vi "Set Data Loop References.vi"(7 "Data Loop Data in":T1, 8 "error in (no error)":errorcluster, 11 "call chain":string[](array[string])) -> (0 "error out":errorcluster, 2 "Data Loop Data out":T1, 3 "VI out":refnum<vi>)   [LabVIEW 2018]
uses:
  Type Defs/Data Loop Data.ctl
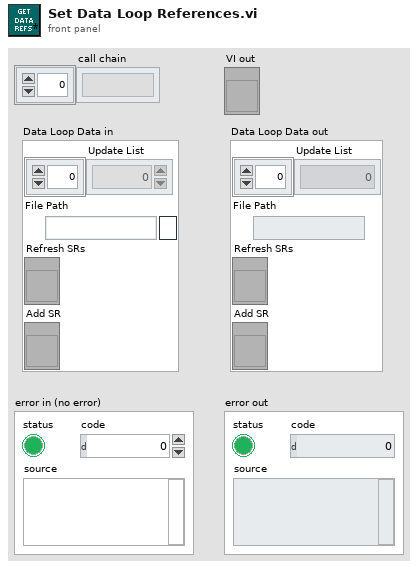
[diagram p1: front panel]
types:
  T1 = typedef "Data Loop Data.ctl" = cluster{"Update List":i32[], "File Path":path, "Refresh SRs":refnum<vi>, "Add SR":refnum<vi>}
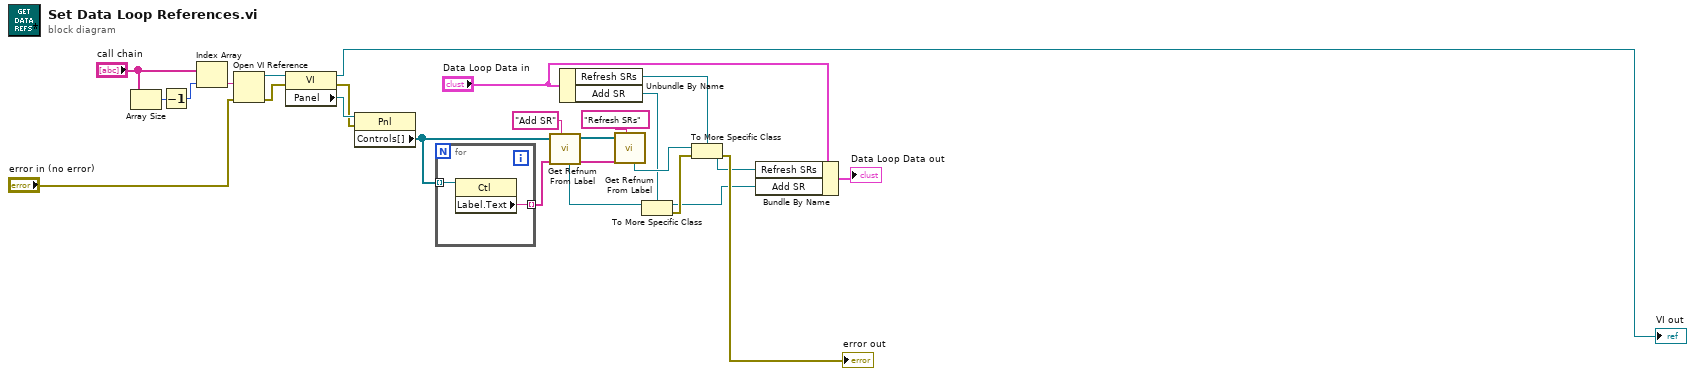
[diagram p0: block diagram]
diagram:
  n1 = Array Size(array="call chain") -> (size(s)=w2:i32)
  n2 = Decrement(x=w2) -> (x-1=w3:i32)
  n3 = Index Array(array="call chain", index=w3) -> (element=w4:string)
  n4 = Open VI Reference(vi path=w4, error in (no error)="error in (no error)") -> (vi reference=w23:refnum<vi>, error out=w16:errorcluster)  [unwired: 4 in]
  n5 = property class="VI"(reference=w23, error in=w16) -> (reference out=→"VI out":refnum<vi>, error out=w17:errorcluster, "Panel"=w18:refnum<vi>)
  n6 = property class="Pnl"(reference=w18, error in=w17) -> ("Controls[]"=w5:refnum<vi>[])  [unwired: 2 out]
  n7 = for {
    tunnel: w5 -> [w28] mode=indexing
    tunnel: [w27] -> w6 mode=indexing
    n8 = property class="Ctl"(reference=w28) -> ("Label.Text"=w27:string)  [unwired: 1 in, 2 out]
  }
  n9 = call "Get Refnum From Label.vi"("label"="Add SR", "label array in"=w6, "controls[] in"=w5) -> ("label array out"=w8:string[], "controls[] out"=w7:refnum<vi>[], "refnum out"=w13:refnum<vi>)  [unwired: 6 in]
  n10 = Unbundle By Name("Data Loop Data in") -> ("Refresh SRs"=w9:refnum<vi>, "Add SR"=w12:refnum<vi>)
  n11 = call "Get Refnum From Label.vi"("label"="Refresh SRs", "label array in"=w8, "controls[] in"=w7) -> ("refnum out"=w15:refnum<vi>)  [unwired: 6 in, 2 out]
  n12 = To More Specific Class(target class=w12, reference=w13) -> (specific class reference=w11:refnum<vi>, error out=w14:errorcluster)  [unwired: 1 in]
  n13 = To More Specific Class(target class=w9, reference=w15, error in=w14) -> (specific class reference=w10:refnum<vi>, error out=→"error out":errorcluster)
  n14 = Bundle By Name(cluster="Data Loop Data in", "Refresh SRs"=w10, "Add SR"=w11) -> (→"Data Loop Data out":T1)
